vi "Configure Demodulation.vi"(7 "Delay Time (6E-6 s)":dbl=6e-06, 8 "error in (no error)":errorcluster, 9 "Speaker Volume (10)":dbl=10.0, 10 "Demodulation Type (0: AM)":i32(ring) items=["AM", "FM"], 11 "VISA resource name":refnum<visa-resource-name>) -> (0 "error out":errorcluster, 3 "VISA resource name out":refnum<visa-resource-name>)   [LabVIEW 2022 SP3, in "Agilent N934X Series.lvlib"]
doc: "Configures the Demodulation of the spectrum analyzer."
uses:
  <instrlib>/Agilent N934X Series/Agilent N934X Series.lvlib
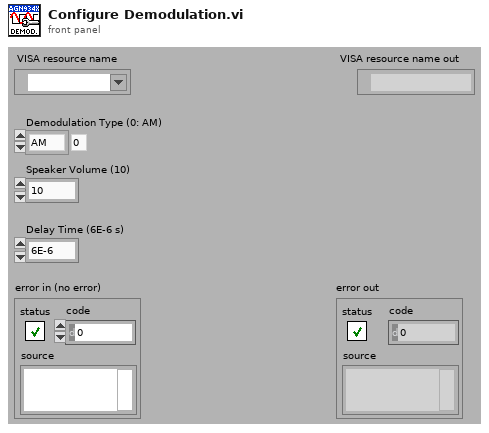
[diagram p1: front panel]
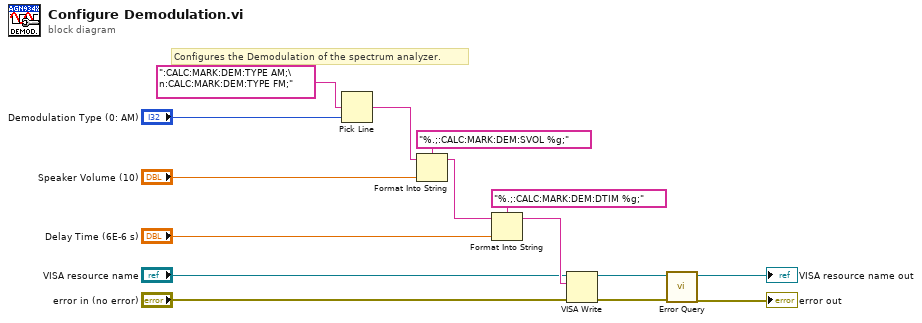
[diagram p0: block diagram]
diagram:
  # "Configures the Demodulation of the spectrum analyzer."
  n1 = Pick Line(multi-line string=":CALC:MARK:DEM:TYPE AM;\n:CALC:MARK:DEM:TYPE FM;", line index="Demodulation Type (0: AM)") -> (output string=w13:string)  [unwired: 1 in]
  n2 = Format Into String(format string="%.;:CALC:MARK:DEM:SVOL %g;", initial string=w13, "Speaker Volume (10)") -> (resulting string=w10:string)  [unwired: 1 in, 1 out]
  n3 = Format Into String(format string="%.;:CALC:MARK:DEM:DTIM %g;", initial string=w10, "Delay Time (6E-6 s)") -> (resulting string=w7:string)  [unwired: 1 in, 1 out]
  n4 = VISA Write(VISA resource name="VISA resource name", write buffer=w7, error in (no error)="error in (no error)") -> (VISA resource name out=w4:refnum<visa-resource-name>, error out=w3:errorcluster)  [unwired: 1 out]
  n5 = call <instrlib>:"Error Query.vi"("error in (no error)"=w3, "VISA resource name"=w4) -> ("error out"=→"error out":errorcluster, "VISA resource name out"=→"VISA resource name out":refnum<visa-resource-name>)  [unwired: 6 in, 2 out]
